vi "Initialize - Individual Address.vi"(7 "Error in":errorcluster caption="错误输入", 9 "Comm. Config.":T1={"Address"=1, "Baud Rate"=115200, "Parity"=0} caption="通讯设置" {"Parity" items=["无校验", "奇校验", "偶检验", "标记", "空格"]; "Baud Rate" items=["1200"=1200, "2400"=2400, "9600"=9600, "19200"=19200, "38400"=38400, "57600"=57600, "115200"=115200]}, 10 "VISA resource name":refnum<visa-resource-name>="COM1" caption="VISA资源名") -> (0 "Error out":errorcluster caption="错误输出", 2 "Channel":i32 caption="通道", 3 "Serial Master Instance":refnum<class "Modbus Master.lvclass"> caption="串口实例")   [LabVIEW 2023, in "Longer Pump dLSP501 Series.lvlib"]
doc: "This VI passes the addressing information in the instrument decriptor to the Instr Open VI and returns the instrument ID. You must run this VI before using any of the instrument driver VIs for this instrument.\n\nNote:\nOnly one Initialize.vi is required when programming multiple instruments on the same port."
uses:
  <instrlib>/Longer Pump dLSP501 Modbus RTU Series/Longer Pump dLSP501 Series.lvlib
  <vilib>/NI/Modbus Library/API/Master/Modbus Master.lvclass
  <vilib>/NI/Modbus Library/API/Wrapper/Create Serial Master.vi
  <vilib>/NI/Modbus Library/API/Wrapper/API Main.lvlib
panel:
  # "Copyright 2024, Longer Precision Pump Co., Ltd."
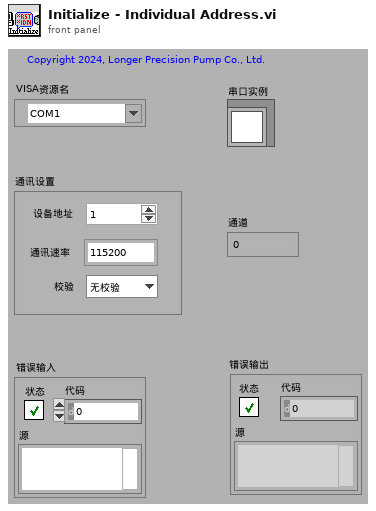
[diagram p1: front panel]
types:
  T1 = cluster{"Address":u8, "Baud Rate":u32, "Parity":u16}
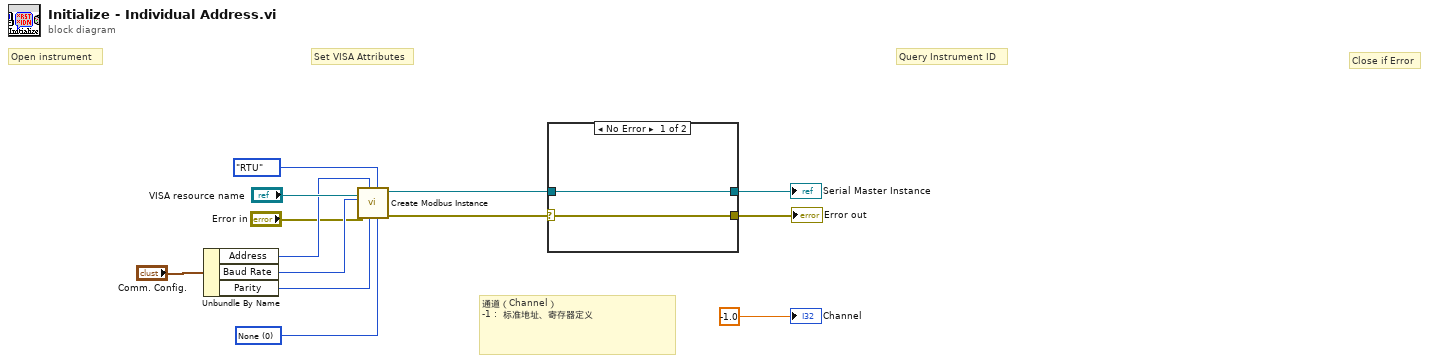
[diagram p0: block diagram]
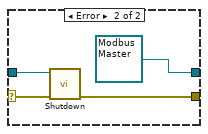
[diagram p2: hidden frame]
diagram:
  w12 = u16 0 items=["None", "XON/XOFF", "RTS/CTS", "XON/XOFF & RTS/CTS", "DTR/DSR", "XON/XOFF & DTR/DSR"] ("flow control (none)")
  # "通道（Channel）\n-1 :  标准地址、寄存器定义"
  # "Set VISA Attributes"
  # "Close if Error"
  # "Query Instrument ID"
  # "Open instrument"
  n1 = Unbundle By Name("Comm. Config.") -> ("Address"=w7:u8, "Baud Rate"=w8:u32, "Parity"=w9:u16)
  n2 = call-poly <vilib>:"Create Modbus Instance.vi"("flow control (none)"=w12, "serial type"=enum16{"RTU", "ASCII"}."RTU", "parity (even)"=w9, "unit ID"=w7, "error in"="Error in", "baud rate"=w8, "VISA resource name"="VISA resource name") -> ("error out"=w6:errorcluster, "serial master instance"=w5:refnum<class "Modbus Master.lvclass">)  [unwired: 3 in]
  n3 = case shown="No Error" w6 {
    selector: w6 -> [w14 w17]
    tunnel: w5 -> [w15 w18]
    tunnel: [w15 refnum<class "Modbus Master.lvclass"> refnum ("serial master instance 2")] -> w4
    tunnel: [w14 w19] -> w2
    frame No Error {
    }
    frame Error {
      n4 = call-dynamic "Shutdown.vi"("error in"=w17, "Modbus master in"=w18) -> ("error out"=w19:errorcluster)  [unwired: 9 in]
    }
  }
  "Serial Master Instance" <- w4
  "Error out" <- w2
  "Channel" <- -1.0 ("Channel")
